vi "HEWH Highest Totalized Volume.vi"(10 "Sub Array End Index in":i32, 11 "Total in":dbl[](array[numeric])) -> (2 "Highest Totalized Volume (gal)":dbl, 3 "Sub Array Out":i32, 5 "Total Sub\nReversed":dbl[](array[numeric]))   [LabVIEW 2023]
panel:
  out "Number of Runs":i32
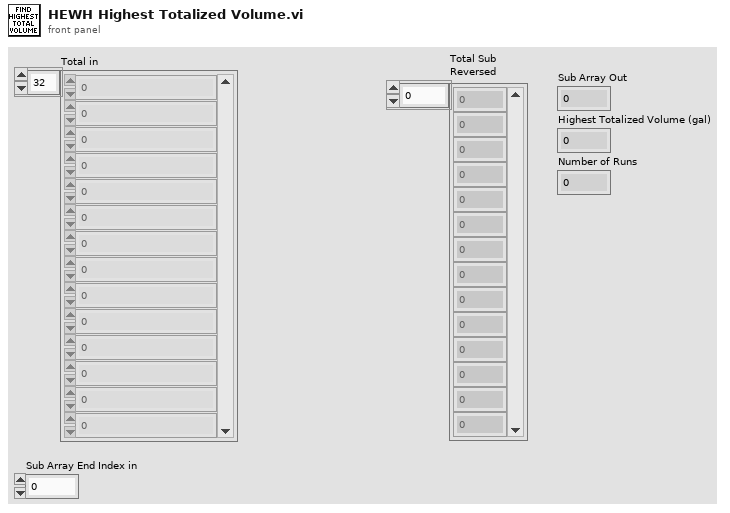
[diagram p1: front panel]
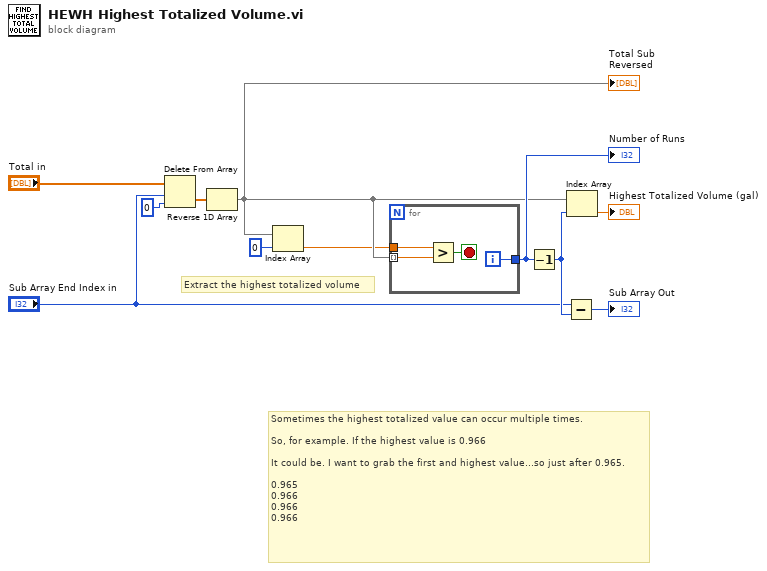
[diagram p0: block diagram]
diagram:
  # "Sometimes the highest totalized value can occur multiple times. \n\nSo, for example. If the highest value is 0.966\n\nIt could be. I want to grab the first and highest value...so just after 0.965.\n\n0.965\n0.966\n0.966\n0.966"
  # "Extract the highest totalized volume"
  n1 = Delete From Array(array="Total in", length="Sub Array End Index in", index=0) -> (deleted portion=w2:dbl[])  [unwired: 1 out]
  n2 = Reverse 1D Array(array=w2) -> (reversed array=w8:dbl[])
  "Total Sub\nReversed" <- w8
  n3 = Index Array(array=w8, index=0) -> (element=w4:dbl)
  n4 = for {
    tunnel: w8 -> [w15] mode=indexing
    tunnel: w4 -> [w14]
    tunnel: [w13] -> w10
    i -> [w13]
    stop <- w12 stop-if-true
    n5 = Greater?(x=w14, y=w15) -> (0:w12:bool)
  }
  "Number of Runs" <- w10
  n6 = Decrement(x=w10) -> (x-1=w11:i32)
  n7 = Subtract(x="Sub Array End Index in", y=w11) -> (x-y=→"Sub Array Out":i32)
  n8 = Index Array(array=w8, index=w11) -> (element=→"Highest Totalized Volume (gal)":dbl)
